vi "Reset.vi"(8 "error in (no error)":errorcluster {"code" format="%.0x"}, 11 "instrument handle":refnum<k15>) -> (0 "error out":errorcluster {"code" format="%.0x"}, 3 "instrument handle out":refnum<k15>)   [LabVIEW 2020, in "Keysight DAQ970.lvlib"]
doc: "Places the instrument in a known state and configures instrument options on which the IVI specific driver depends (for example, enabling/disabling headers). For an IEEE 488.2 instrument, Reset sends the command string *RST to the instrument."
uses:
  Keysight DAQ970.lvlib
  KtDAQ970.dll
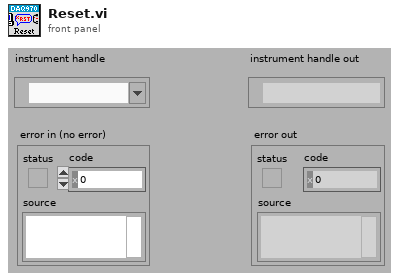
[diagram p1: front panel]
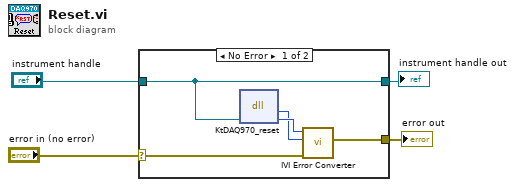
[diagram p0: block diagram]
diagram:
  n1 = case shown="No Error" "error in (no error)" {
    selector: "error in (no error)" -> [w6 w10]
    tunnel: [w8 w10] -> w4
    tunnel: "instrument handle" -> [w5 w11]
    tunnel: [w5 w11] -> w1
    frame No Error {
      n2 = dll-call lib="KtDAQ970**.dll" fn="KtDAQ970_reset" ("LabVIEW:IviDmm_reset")("instrument handle"=w5) -> ("Status"=w7:i32, "instrument handle"=w9:u32)  [unwired: 3 in, 2 out]
      n3 = call "IVI Error Converter.vi"("error in (no error)"=w6, "IVI error code (0)"=w7, "instrument handle"=w9) -> ("error out"=w8:errorcluster)  [unwired: 7 in, 1 out]
    }
    frame Error {
    }
  }
  "error out" <- w4
  "instrument handle out" <- w1
